vi "findast.vi"(3 "ImgAstrom IN":T1 {"CRVAL" format="%.6g"; "CD" format="%_7g"}, 8 "Y":dbl[](array[numeric]), 9 "X":dbl[](array[numeric]), 10 "DEC":dbl[](array[numeric]), 11 "RA":dbl[](array[numeric])) -> (0 "ImgAstrom OUT":T1 {"CRVAL" format="%.6g"; "CD" format="%_7g"}, 4 "Accepted?":bool)   [LabVIEW 2019]
uses:
  <vilib>/Utility/file.llb/Write To Spreadsheet File (DBL).vi
  <vilib>/Utility/file.llb/Read From Spreadsheet File (DBL).vi
panel:
  in  "idl_dir":path=path "C:/UdeM/BonOMM-10/IDL/coords.dat"
  out "standard error":string
  out "standard output":string
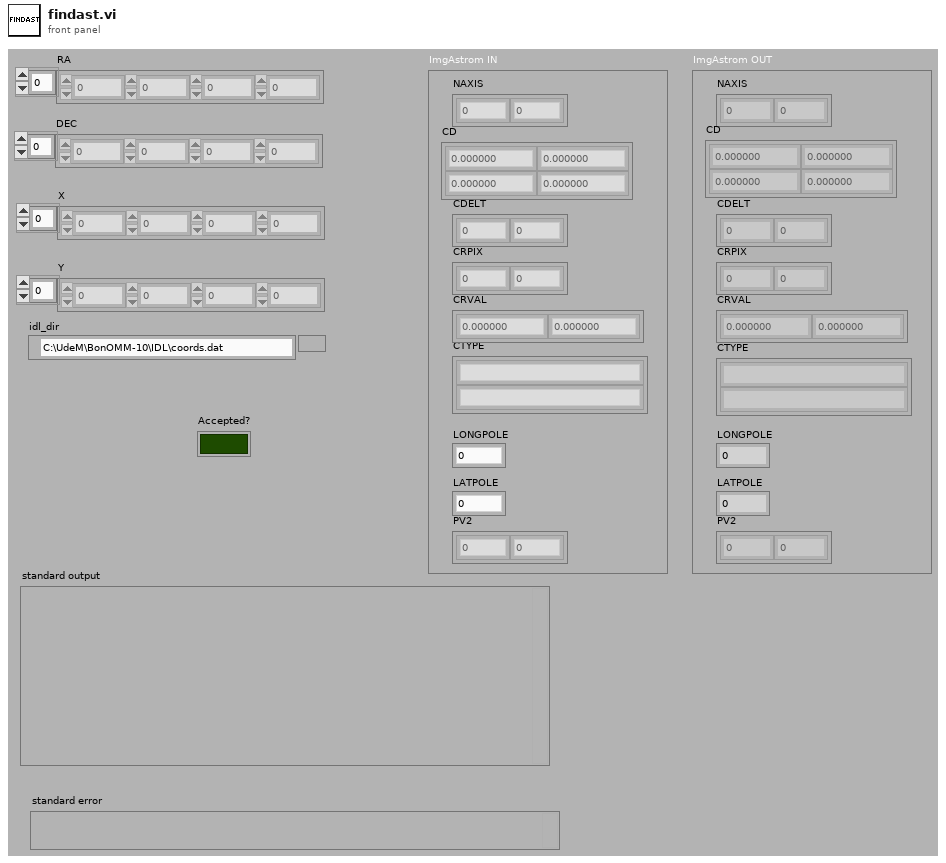
[diagram p1: front panel]
types:
  T1 = cluster{"NAXIS":dbl[], "CD":dbl[][], "CDELT":dbl[], "CRPIX":dbl[], "CTYPE":string[], "CRVAL":dbl[], "LONGPOLE":dbl, "LATPOLE":dbl, "PV2":dbl[]}
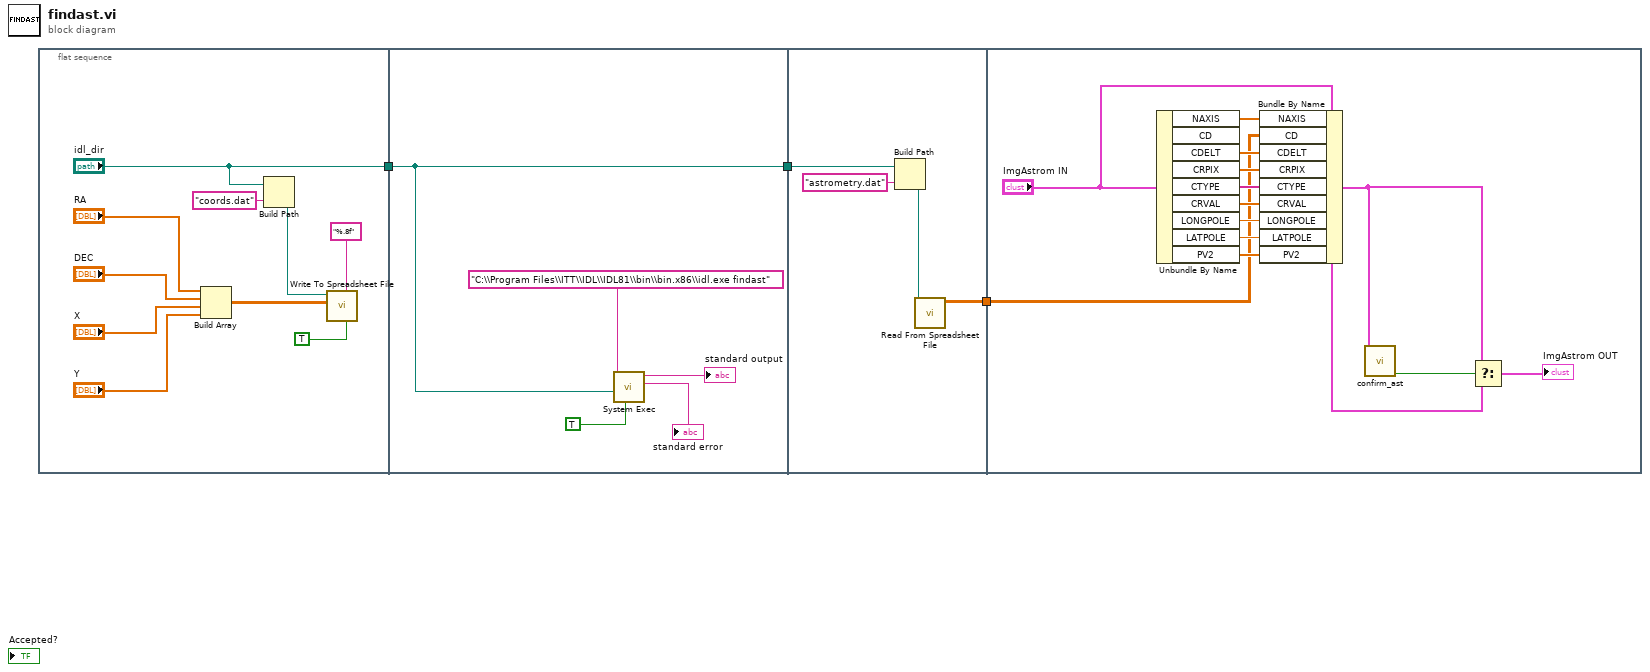
[diagram p0: block diagram]
diagram:
  n1 = flat-sequence {
    tunnel: ["idl_dir"] -> w3
    tunnel: w3 -> [w14]
    tunnel: [w14] -> w2
    tunnel: w2 -> [w20]
    tunnel: [w19] -> w1
    tunnel: w1 -> [w27]
    frame #0 {
      n2 = Build Array("RA", "DEC", "X", "Y") -> (w9:dbl[][])
      n3 = Build Path(base path="idl_dir", name or relative path="coords.dat") -> (appended path=w4:path)
      n4 = call-poly <vilib>:"Write To Spreadsheet File.vi"("transpose? (no:F)"=TRUE, "format (%.3f)"="%.8f", "2D data"=w9, "file path (dialog if empty)"=w4) -> ()  [unwired: 4 in, 1 out]
    }
    frame #1 {
      n5 = call <vilib>:"System Exec.vi"("run minimized? (F)"=TRUE, "working directory"=w14, "command line"="C:\\Program Files\\ITT\\IDL\\IDL81\\bin\\bin.x86\\idl.exe findast") -> ("standard error"=→"standard error":string, "standard output"=→"standard output":string)  [unwired: 5 in, 2 out]
    }
    frame #2 {
      n6 = Build Path(base path=w20, name or relative path="astrometry.dat") -> (appended path=w22:path)
      n7 = call-poly <vilib>:"Read From Spreadsheet File.vi"("file path (dialog if empty)"=w22) -> ("all rows"=w19:dbl[][])  [unwired: 6 in, 4 out]
    }
    frame #3 {
      n8 = Unbundle By Name("ImgAstrom IN") -> ("NAXIS"=w35:dbl[], "CDELT"=w34:dbl[], "CRPIX"=w33:dbl[], "CTYPE"=w32:string[], "CRVAL"=w31:dbl[], "LONGPOLE"=w30:dbl, "LATPOLE"=w29:dbl, "PV2"=w28:dbl[])  [unwired: 1 out]
      n9 = Bundle By Name(cluster="ImgAstrom IN", "NAXIS"=w35, "CD"=w27, "CDELT"=w34, "CRPIX"=w33, "CTYPE"=w32, "CRVAL"=w31, "LONGPOLE"=w30, "LATPOLE"=w29, "PV2"=w28) -> (w24:T1)
      n10 = call "confirm_ast.vi"("ImgAstrom IN"=w24) -> ("Accepted?"=w26:bool)  [unwired: 9 in, 1 out]
      n11 = Select(t=w24, s=w26, f="ImgAstrom IN") -> (s? t:f=→"ImgAstrom OUT":T1)
    }
  }
